vi "Set Averaging.vi"(8 "error in (no error)":errorcluster, 9 "Averaging":i16(slide) scale=0.0..1.0, 11 "VISA resource name":refnum<visa-resource-name>) -> (0 "error out":errorcluster, 3 "VISA resource name out":refnum<visa-resource-name>)   [LabVIEW 2017]
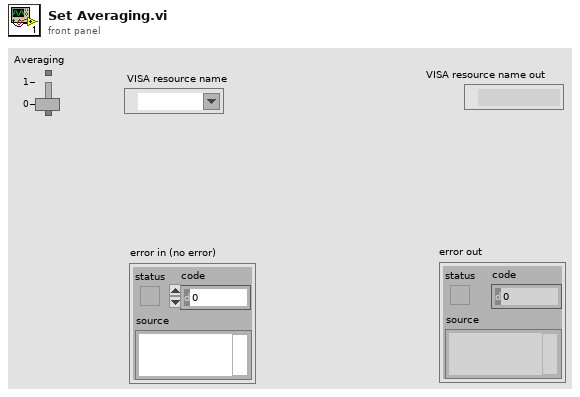
[diagram p1: front panel]
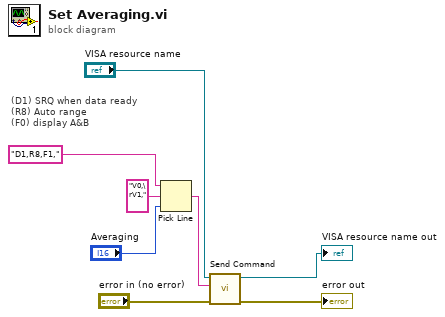
[diagram p0: block diagram]
diagram:
  # "(D1) SRQ when data ready\n(R8) Auto range\n(F0) display A&B"
  n1 = Pick Line(string ("")="D1,R8,F1,", multi-line string="V0,\rV1,", line index="Averaging") -> (output string=w1:string)
  n2 = call "Send Command.vi"("error in (no error)"="error in (no error)", "write buffer"=w1, "VISA resource name"="VISA resource name") -> ("error out"=→"error out":errorcluster, "VISA resource name out"=→"VISA resource name out":refnum<visa-resource-name>)  [unwired: 7 in]
